vi "main2.vi"() -> ()   [LabVIEW 2018]
uses:
  <vilib>/Platform/TimedLoop/XDataNode/timing_clust.ctl
  <vilib>/Platform/TimedLoop/XDataNode/nitl_modes.ctl
  <vilib>/Platform/TimedLoop/XDataNode/wakeup.ctl
  <vilib>/rvi/Emulation/niFpgaSctlEmulationGetInTimedLoop.vi
  <vilib>/rvi/Emulation/niFpgaEmulationReportErrorSimple.vi
  <vilib>/rvi/Emulation/niFpgaGetClockAttributes.vi
  <vilib>/rvi/Emulation/niFpgaCriticalErrorInLSC.vi
  <vilib>/rvi/Emulation/niFpgaProcessEmulError.vi
  <vilib>/Platform/TimedLoop/XDataNode/XDataNode.xnode
  <vilib>/Platform/TimedLoop/XDataNode/XDNodeRunTimeDep.lvlib
panel:
  out "t_cell_max":fxp<+/-,32,16>
  out "t_cell_min":fxp<+/-,32,16>
  out "p_4_max":fxp<+/-,32,16>
  out "p_4_min":fxp<+/-,32,16>
  out "p_3_max":fxp<+/-,32,16>
  out "p_3_min":fxp<+/-,32,16>
  out "p_2_max":fxp<+/-,32,16>
  out "p_2_min":fxp<+/-,32,16>
  out "p_1_max":fxp<+/-,32,16>
  out "p_1_min":fxp<+/-,32,16>
  out "t_pistions_max":fxp<+/-,32,16>
  out "t_pistions_min":fxp<+/-,32,16>
  out "t_pneum_tank_max":fxp<+/-,32,16>
  out "t_pneum_tank_min":fxp<+/-,32,16>
  out "t_res_bat_max":fxp<+/-,32,16>
  out "t_res_bat_min":fxp<+/-,32,16>
  out "t_prime_bat_2_max":fxp<+/-,32,16>
  out "t_prime_bat_2_min":fxp<+/-,32,16>
  out "t_prime_bat_1_max":fxp<+/-,32,16>
  out "t_prime_bat_1_min":fxp<+/-,32,16>
  in  "new_val":fxp<+/-,32,16>
  in  "threshold_write_val":fxp<+/-,32,16>
  in  "threshold_write_latch":bool
  in  "threshold_write_index":u8
  in  "stop":bool
  in  "fxp32_16":fxp<+/-,32,16>
  out "fault_t_pistons":bool
  out "fault_t_pneum_tank":bool
  out "fault_t_res_bat":bool
  out "fault_t_prime_bat_2":bool
  out "fault_t_prime_bat_1":bool
  in  "prim_bat_3":bool
  in  "prim_bat_2":bool
  in  "prim_bat_1":bool
  out "t_pistons":i32
  out "t_pneum_tank":i32
  out "t_res_bat":i32
  out "t_prime_bat_2":i32
  out "t_prime_bat_1":i32
  out "count_laser_l":u16
  out "count_laser_r":u16
  out "count_light_bl":u16
  out "count_light_br":u16
  out "count_light_fl":u16
  out "count_light_fr":u16
  out "voltage_3":i32
  out "voltage_2":i32
  out "voltage_1":i32
  out "current_3":i32
  out "currents_2":i32
  out "current_1":i32
  in  "solenoid_3":bool
  in  "solenoid_2":bool
  in  "solenoid_1":bool
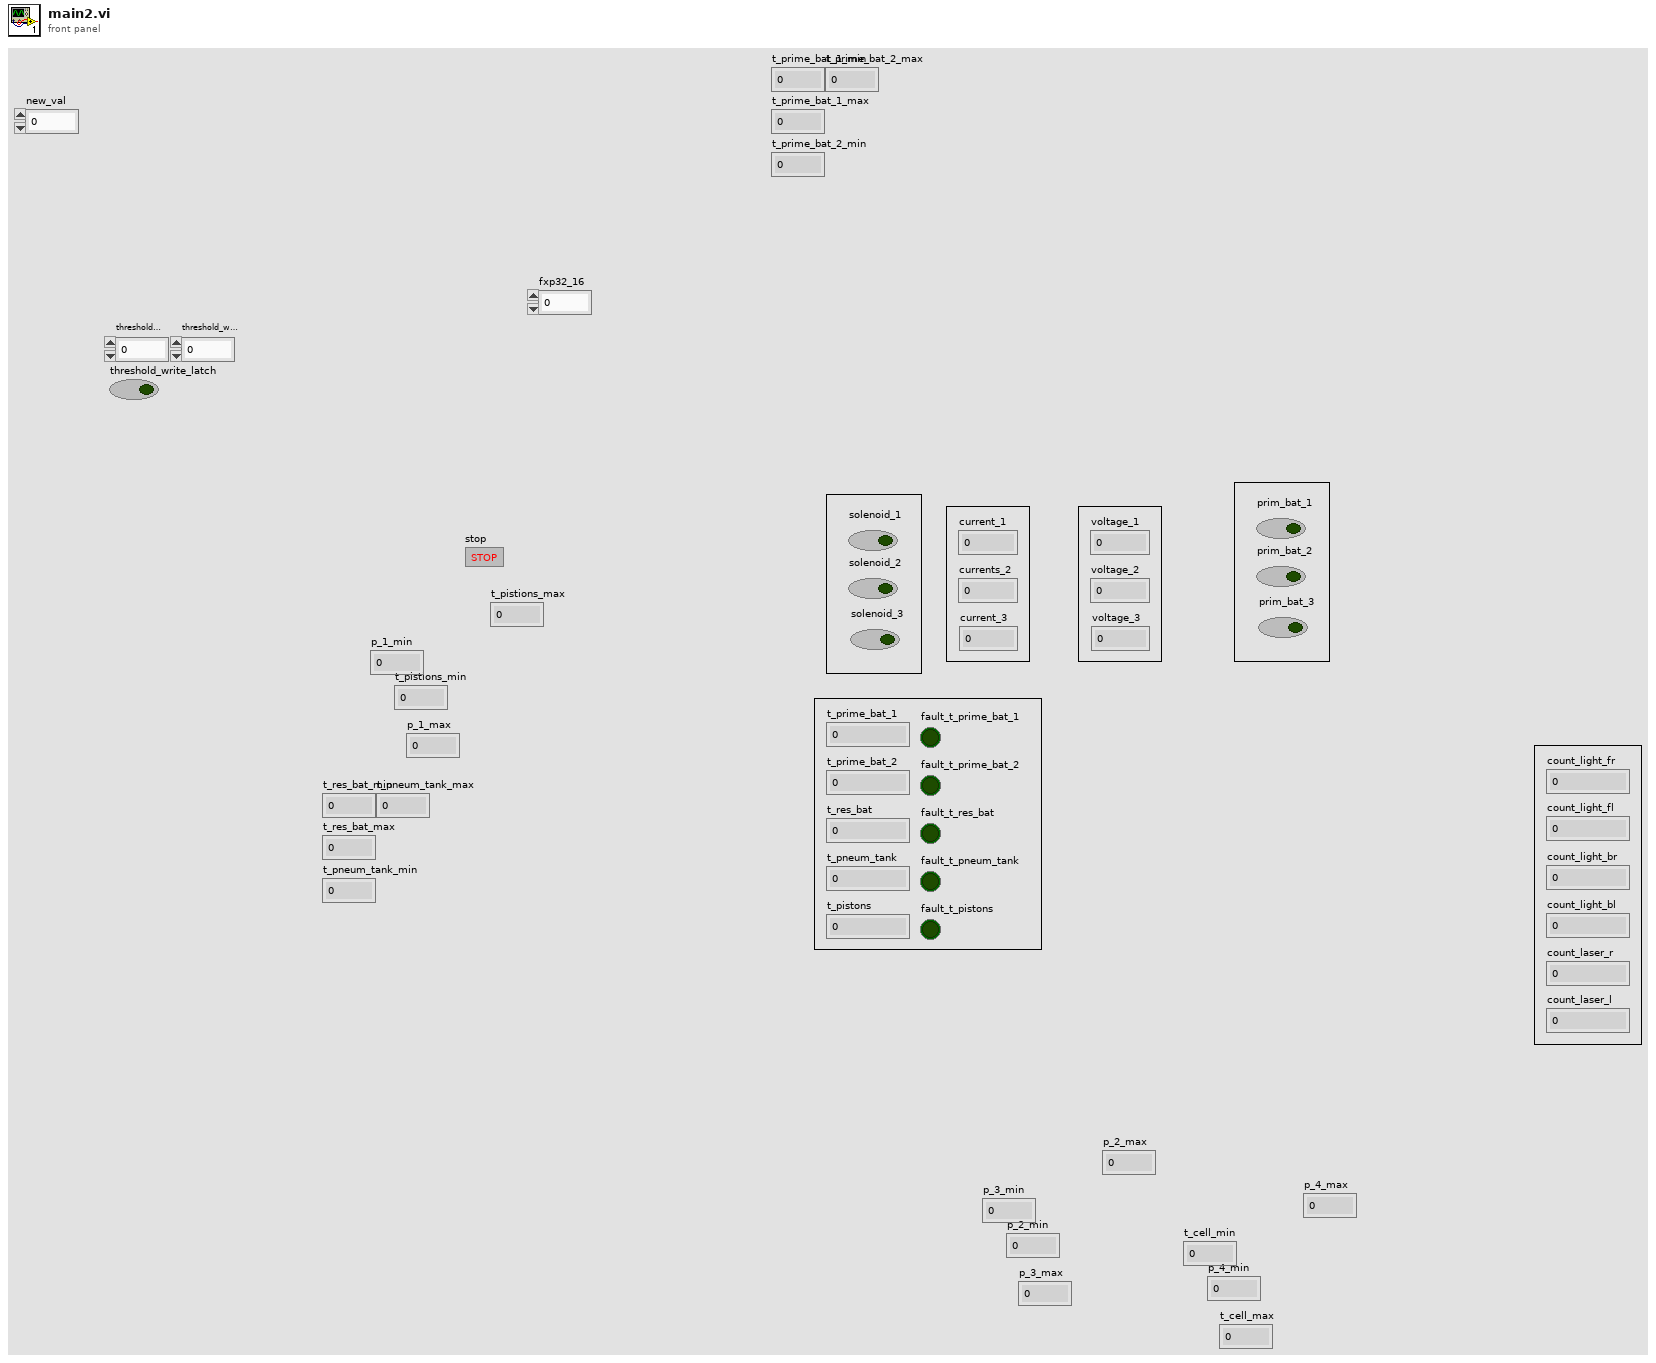
[diagram p1: front panel]
types:
  T1 = typedef "XDNodeRunTimeDep.lvlib/timing_clust.ctl" = cluster{"Expected End [f-1]":u64, "Actual End [f-1]":u64, "Finished Late? [f-1]":bool, "Expected End [i-1]":u64, "Actual End [i-1]":u64, "Finished Late? [i-1]":bool, "Expected Start [i]":u64, "Actual Start [i]":u64, "Expected Start [f]":u64, "Actual Start [f]":u64, "Source Name":string, "Structure Name":string, "Period":i64, "Deadline":i64, "Offset":i64, "Start":i64, "Priority":i32, "Timeout":i32, "Mode":T2, "Wakeup Reason":T3, "Error":errorcluster, "Source Type":string, "Secondary Source Type":string, "Global End Time":u64, "Global Start Time":u64, "Frame Duration":u64, "Iteration Duration":u64, "Assigned CPU":i32, "I/O Scan Engine Mode":u32}
  T2 = typedef "XDNodeRunTimeDep.lvlib/nitl_modes.ctl" = enum32{"No Change", "Process missed periods, maintain original phase", "Discard missed periods, maintain original phase", "Process missed periods, ignore original phase", "Discard missed periods, ignore original phase"}
  T3 = typedef "XDNodeRunTimeDep.lvlib/wakeup.ctl" = enum32{"Normal", "Aborted", "Asynchronous wakeup", "Timing source error", "Timed loop error", "Timeout"}
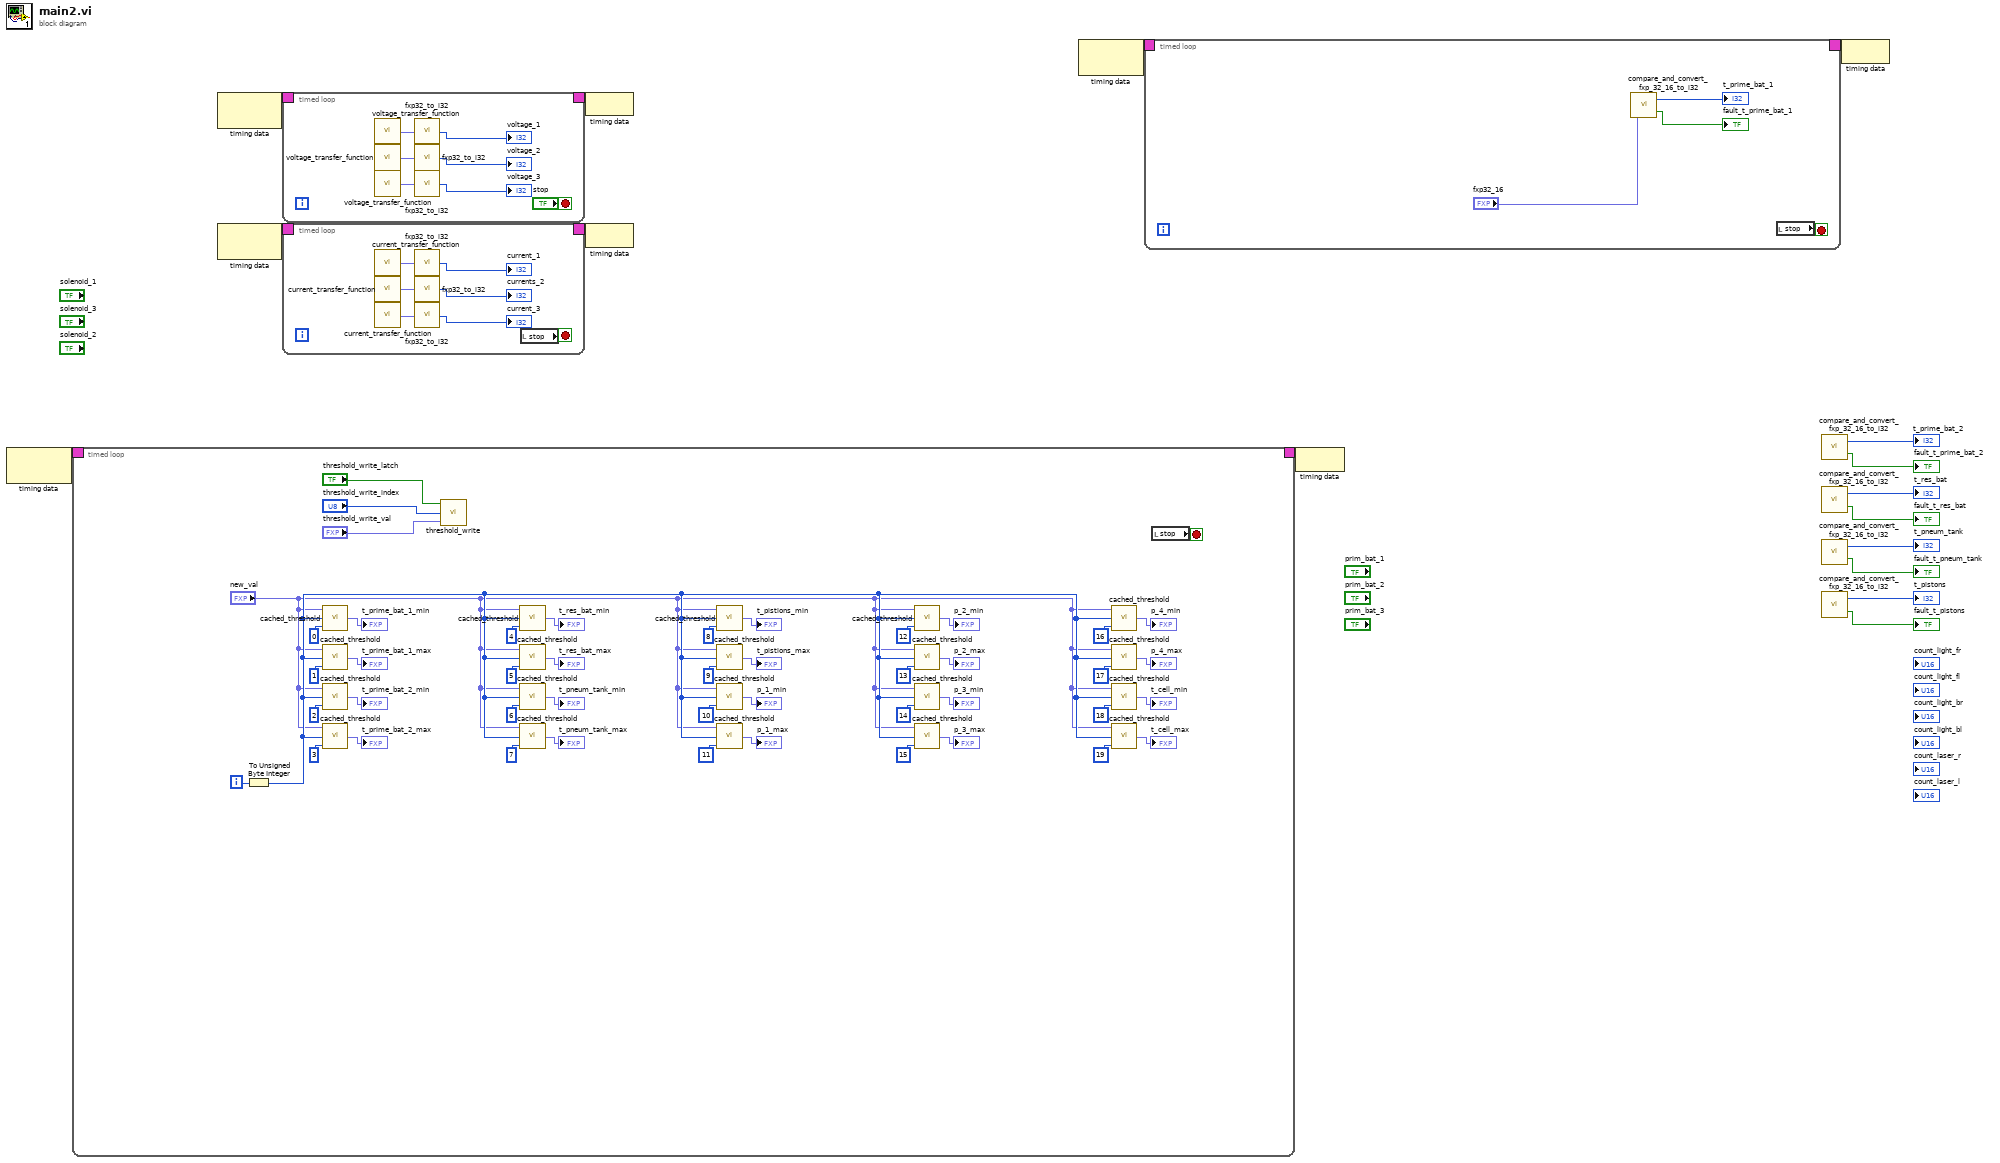
[diagram p0: block diagram]
diagram:
  n1 = node-c288() -> (w2:T1)  [unwired: 1 in]
  n2 = timed-loop {
    timing: w2 -> [_]
    timing-out: [_] -> w1
    i -> [w62]
    stop <- w63 stop-if-true
    n3 = To Unsigned Byte Integer(number=w62) -> (unsigned 8bit integer=w18:u8)
    n4 = call "cached_threshold.vi"("index"=u8 0, "cur_index"=w18, "new_val"="new_val") -> ("$_val"=→"t_prime_bat_1_min":fxp<+/-,32,16>)
    n5 = call "cached_threshold.vi"("index"=u8 1, "cur_index"=w18, "new_val"="new_val") -> ("$_val"=→"t_prime_bat_1_max":fxp<+/-,32,16>)
    n6 = call "cached_threshold.vi"("index"=u8 2, "cur_index"=w18, "new_val"="new_val") -> ("$_val"=→"t_prime_bat_2_min":fxp<+/-,32,16>)
    n7 = call "cached_threshold.vi"("index"=u8 3, "cur_index"=w18, "new_val"="new_val") -> ("$_val"=→"t_prime_bat_2_max":fxp<+/-,32,16>)
    n8 = call "threshold_write.vi"("new_value"="threshold_write_val", "index"="threshold_write_index", "latch"="threshold_write_latch") -> ()  [unwired: 1 in]
    n9 = call "cached_threshold.vi"("index"=u8 4, "cur_index"=w18, "new_val"="new_val") -> ("$_val"=→"t_res_bat_min":fxp<+/-,32,16>)
    n10 = call "cached_threshold.vi"("index"=u8 5, "cur_index"=w18, "new_val"="new_val") -> ("$_val"=→"t_res_bat_max":fxp<+/-,32,16>)
    n11 = call "cached_threshold.vi"("index"=u8 6, "cur_index"=w18, "new_val"="new_val") -> ("$_val"=→"t_pneum_tank_min":fxp<+/-,32,16>)
    n12 = call "cached_threshold.vi"("index"=u8 7, "cur_index"=w18, "new_val"="new_val") -> ("$_val"=→"t_pneum_tank_max":fxp<+/-,32,16>)
    n13 = call "cached_threshold.vi"("index"=u8 8, "cur_index"=w18, "new_val"="new_val") -> ("$_val"=→"t_pistions_min":fxp<+/-,32,16>)
    n14 = call "cached_threshold.vi"("index"=u8 9, "cur_index"=w18, "new_val"="new_val") -> ("$_val"=→"t_pistions_max":fxp<+/-,32,16>)
    n15 = call "cached_threshold.vi"("index"=u8 10, "cur_index"=w18, "new_val"="new_val") -> ("$_val"=→"p_1_min":fxp<+/-,32,16>)
    n16 = call "cached_threshold.vi"("index"=u8 11, "cur_index"=w18, "new_val"="new_val") -> ("$_val"=→"p_1_max":fxp<+/-,32,16>)
    n17 = call "cached_threshold.vi"("index"=u8 12, "cur_index"=w18, "new_val"="new_val") -> ("$_val"=→"p_2_min":fxp<+/-,32,16>)
    n18 = call "cached_threshold.vi"("index"=u8 13, "cur_index"=w18, "new_val"="new_val") -> ("$_val"=→"p_2_max":fxp<+/-,32,16>)
    n19 = call "cached_threshold.vi"("index"=u8 14, "cur_index"=w18, "new_val"="new_val") -> ("$_val"=→"p_3_min":fxp<+/-,32,16>)
    n20 = call "cached_threshold.vi"("index"=u8 15, "cur_index"=w18, "new_val"="new_val") -> ("$_val"=→"p_3_max":fxp<+/-,32,16>)
    n21 = call "cached_threshold.vi"("index"=u8 16, "cur_index"=w18, "new_val"="new_val") -> ("$_val"=→"p_4_min":fxp<+/-,32,16>)
    n22 = call "cached_threshold.vi"("index"=u8 17, "cur_index"=w18, "new_val"="new_val") -> ("$_val"=→"p_4_max":fxp<+/-,32,16>)
    n23 = call "cached_threshold.vi"("index"=u8 18, "cur_index"=w18, "new_val"="new_val") -> ("$_val"=→"t_cell_min":fxp<+/-,32,16>)
    n24 = call "cached_threshold.vi"("index"=u8 19, "cur_index"=w18, "new_val"="new_val") -> ("$_val"=→"t_cell_max":fxp<+/-,32,16>)
    n25 = local read "stop"() -> (w63:bool)
  }
  n26 = node-c288() -> (w8:T1)  [unwired: 1 in]
  n27 = node-c288() -> (w6:T1)  [unwired: 1 in]
  n28 = timed-loop {
    timing: w8 -> [_]
    timing-out: [_] -> w7
    stop <- "stop" stop-if-true
    n29 = call "voltage_transfer_function.vi"() -> ("V"=w69:fxp<+/-,32,16>)  [unwired: 1 in]
    n30 = call "voltage_transfer_function.vi"() -> ("V"=w68:fxp<+/-,32,16>)  [unwired: 1 in]
    n31 = call "voltage_transfer_function.vi"() -> ("V"=w67:fxp<+/-,32,16>)  [unwired: 1 in]
    n32 = call "fxp32_to_i32.vi"("fxp32_16"=w69) -> ("32bit integer"=→"voltage_1":i32)
    n33 = call "fxp32_to_i32.vi"("fxp32_16"=w68) -> ("32bit integer"=→"voltage_2":i32)
    n34 = call "fxp32_to_i32.vi"("fxp32_16"=w67) -> ("32bit integer"=→"voltage_3":i32)
  }
  n35 = timed-loop {
    timing: w6 -> [_]
    timing-out: [_] -> w5
    stop <- w75 stop-if-true
    n36 = call "current_transfer_function.vi"() -> ("I"=w78:fxp<+/-,32,16>)  [unwired: 1 in]
    n37 = call "current_transfer_function.vi"() -> ("I"=w77:fxp<+/-,32,16>)  [unwired: 1 in]
    n38 = call "current_transfer_function.vi"() -> ("I"=w76:fxp<+/-,32,16>)  [unwired: 1 in]
    n39 = call "fxp32_to_i32.vi"("fxp32_16"=w78) -> ("32bit integer"=→"current_1":i32)
    n40 = call "fxp32_to_i32.vi"("fxp32_16"=w77) -> ("32bit integer"=→"currents_2":i32)
    n41 = call "fxp32_to_i32.vi"("fxp32_16"=w76) -> ("32bit integer"=→"current_3":i32)
    n42 = local read "stop"() -> (w75:bool)
  }
  n43 = node-c288(w7) -> ()
  n44 = node-c288(w5) -> ()
  n45 = node-c288() -> (w4:T1)  [unwired: 1 in]
  n46 = timed-loop {
    timing: w4 -> [_]
    timing-out: [_] -> w3
    stop <- w84 stop-if-true
    n47 = call "compare_and_convert_fxp_32_16_to_i32.vi"("fxp32_16"="fxp32_16") -> ("out_of_range"=→"fault_t_prime_bat_1":bool, "32bit integer"=→"t_prime_bat_1":i32)  [unwired: 2 in]
    n48 = local read "stop"() -> (w84:bool)
  }
  n49 = node-c288(w1) -> ()
  n50 = call "compare_and_convert_fxp_32_16_to_i32.vi"() -> ("out_of_range"=→"fault_t_prime_bat_2":bool, "32bit integer"=→"t_prime_bat_2":i32)  [unwired: 3 in]
  n51 = call "compare_and_convert_fxp_32_16_to_i32.vi"() -> ("out_of_range"=→"fault_t_res_bat":bool, "32bit integer"=→"t_res_bat":i32)  [unwired: 3 in]
  n52 = call "compare_and_convert_fxp_32_16_to_i32.vi"() -> ("out_of_range"=→"fault_t_pneum_tank":bool, "32bit integer"=→"t_pneum_tank":i32)  [unwired: 3 in]
  n53 = call "compare_and_convert_fxp_32_16_to_i32.vi"() -> ("out_of_range"=→"fault_t_pistons":bool, "32bit integer"=→"t_pistons":i32)  [unwired: 3 in]
  n54 = node-c288(w3) -> ()
